vi "Write Pin Register.vi"(10 "state":u8, 11 "DIO in":refnum<class "Digital IO.lvclass">) -> (3 "done":bool)   [LabVIEW 2017, in "Digital IO.lvlib" / "Digital IO.lvclass"]
uses:
  Digital IO.lvclass
  Digital IO.lvclass/Digital IO.ctl
  <vilib>/rvi/DataTransferAndStorage/Container/Common/niFpgaContainerExecOnDevCompGetState.vi
  <vilib>/rvi/Emulation/niFpgaEmulationIsFPGAContextNoSignature.vi
  <vilib>/rvi/DataTransferAndStorage/Container/Common/niFpgaContainerGetUniqueNameForEmu.vi
  <vilib>/rvi/eio/common/nirviEmuReportErrorAndStop.vi
  <vilib>/rvi/Emulation/niFpgaSctlEmulationGetInTimedLoop.vi
  <vilib>/rvi/Emulation/niFpgaProcessEmulError.vi
  <vilib>/rvi/DataTransferAndStorage/Container/XNode/niFpgaContainer.xnode
  <vilib>/rvi/DataTransferAndStorage/Handshake/Emulation/niFpgaHandshakeEmulationRefIn.vi
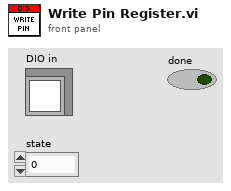
[diagram p1: front panel]
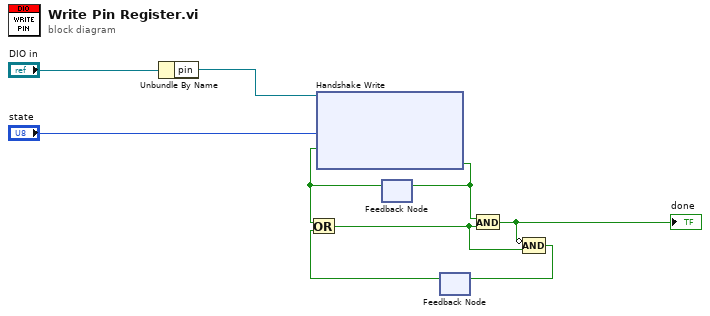
[diagram p0: block diagram]
diagram:
  n1 = Unbundle By Name("DIO in") -> ("pin"=w5:refnum<k21>)
  n2 = feedback #1() -> (w3:bool)  [unwired: 1 in]
  n3 = xnode ("Handshake Write")("Data"="state", "Input Valid"=w3, "Handshake In"=w5) -> ("Ready for Input"=w2:bool)  [unwired: 1 out]
  n4 = feedback-in #1(w2) -> ()
  n5 = feedback #2() -> (w9:bool)  [unwired: 1 in]
  n6 = Or(x=w3, y=w9) -> (x .or. y?=w7:bool)
  n7 = And(x=w2, y=w7) -> (x .and. y?=w6:bool)
  "done" <- w6
  n8 = Compound Arithmetic op=AND(invert w6, w7) -> (w8:bool)
  n9 = feedback-in #2(w8) -> ()
